vi "GenerateCode.vi"(1 "Terms":T1[](array[typedef]), 3 "Diagram":refnum<vi>, 5 "XRef":refnum<vi>, 6 "State In":T4) -> (0 "Generated Code?":bool, 2 "State Out":T4, 4 "Reply":string[](array[string]))   [LabVIEW 2015, in "Async.xnode"]
doc: "This ability VI is called when it is time to define the execution behavior of your XNode via LabVIEW's scripting API. This VI is only called when you have previously informed LabVIEW that you need to script through a GenerateCode reply. Diagram is a reference to a diagram of a temporary VI. This diagram contains exactly one front panel terminal for each terminal of your XNode. Terms is an array of pairs of Term IDs and terminal references. LabVIEW will copy code scripted into this diagram into your XNode and connect everything to the correct terminals. The front panel terminals that are on this diagram are special in that they can only be on the top level diagram.\n \n Generate Code? is used to tell LabVIEW whether or not you want to copy the scripted diagram over. If there is an error and you wish not to commit the changes, then the old XNode behavior will be left unchanged. If you set Generate Code? to false, then this VI will be called again next time type propagation is run. Otherwise, it will not be called until you indicate that it should be through the reply on another ability VI.\n \n Because the diagram you are scripting into is separate from the VI containing the XNode instance, type propagation and the data manager will run on the temporary VI after each scripting call.\n \n You should not use the Copy scripting method to move code into the temporary VI. This will adversely affect the user's clipboard. You should use the Move scripting method instead.\n\nDefault behavior: None.\n\nThis ability does not provide UI and OS messages are not handled.\n\nSee also: ModifyCode"
uses:
  Async.xnode
  State.ctl
  <vilib>/Utility/miscctls.llb/LVRectTypeDef.ctl
  <vilib>/picture/picture.llb/imagedata.ctl
  <vilib>/XNodeSupport/XNodeTermIDPair.ctl
  <vilib>/XNodeSupport/XNodeTermRef.ctl
  <vilib>/XNodeSupport/XNodeString.ctl
  <vilib>/Erdos Miller/LV-Scripting/LV-Scripting.lvlib
  <vilib>/Erdos Miller/LV-VI/LV-VI.lvlib
  <vilib>/XNodeSupport/NI_XNodeSupport.lvlib
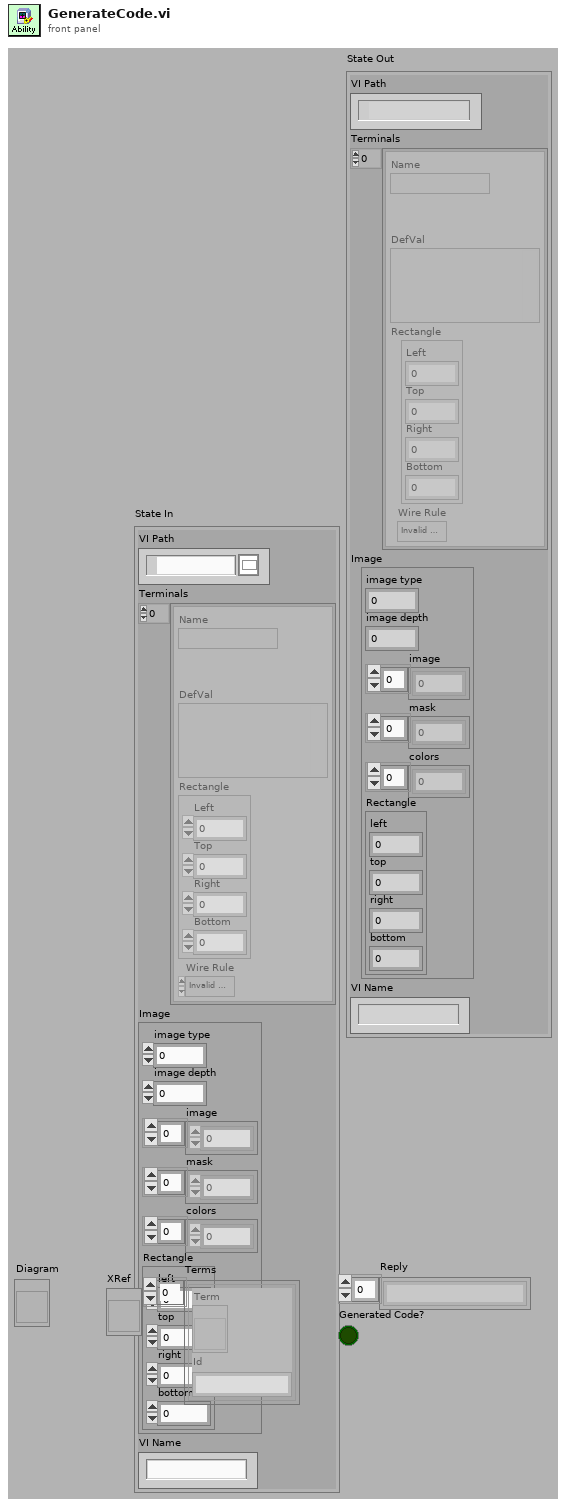
[diagram p1: front panel]
types:
  T1 = typedef "NI_XNodeSupport.lvlib/XNodeTermIDPair.ctl" = cluster{"Term":T2, "Id":T3}
  T2 = typedef "NI_XNodeSupport.lvlib/XNodeTermRef.ctl" = refnum<vi>
  T3 = typedef "NI_XNodeSupport.lvlib/XNodeString.ctl" = string
  T4 = typedef "Async.xnode/State.ctl" = cluster{"VI Path":path, "Terminals":cluster{"Name":string, "DefVal":variant, "Rectangle":T5, "Wire Rule":enum16{"Invalid Wire Rule", "Required", "Recommended", "Optional", "Dynamic Dispatch"}}[], "Image":T6, "VI Name":string}
  T5 = typedef "LVRectTypeDef.ctl" = cluster{"Left":i16, "Top":i16, "Right":i16, "Bottom":i16}
  T6 = typedef "imagedata.ctl" = cluster{"image type":i32, "image depth":i32, "image":u8[], "mask":u8[], "colors":u32[], "Rectangle":cluster{"left":i16, "top":i16, "right":i16, "bottom":i16}}
  T7 = cluster{"Name":string, "DefVal":variant, "Rectangle":T5, "Wire Rule":enum16{"Invalid Wire Rule", "Required", "Recommended", "Optional", "Dynamic Dispatch"}}[]
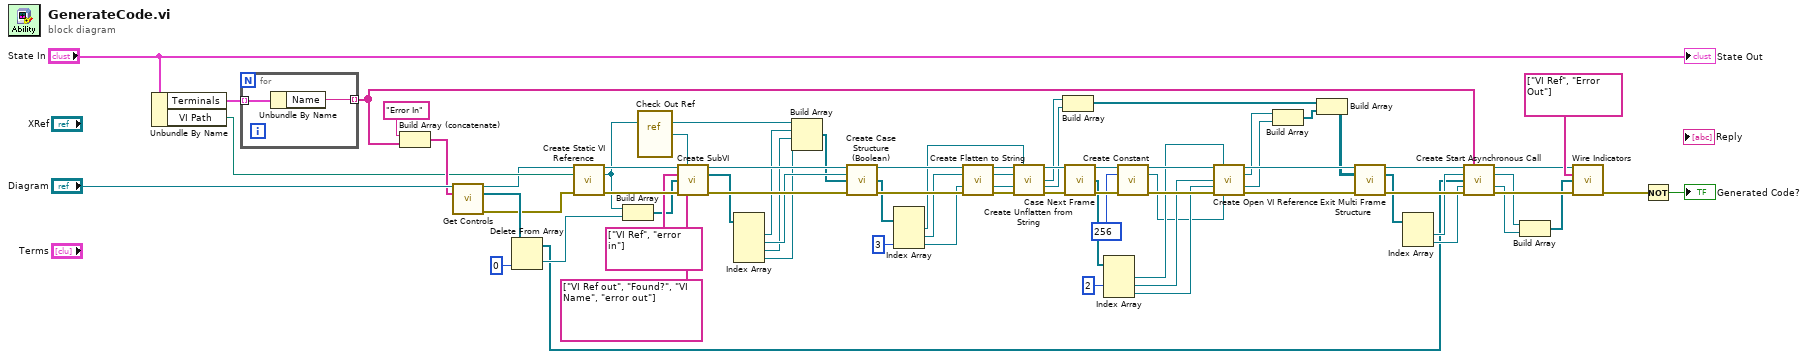
[diagram p0: block diagram]
diagram:
  n1 = Unbundle By Name("State In") -> ("Terminals"=w72:T7, "VI Path"=w67:path)
  n2 = for {
    tunnel: w72 -> [w76] mode=indexing
    tunnel: [w75] -> w4 mode=indexing
    n3 = Unbundle By Name(w76) -> ("Name"=w75:string)
  }
  n4 = Build Array (concatenate)("Error In" ("string"), w4) -> (w70:string[])
  n5 = call <vilib>:"Get Controls.vi"("Diagram in"="Diagram", "Control Names"=w70) -> ("Diagram out"=w66:refnum<vi>, "Control Terminals"=w69:refnum<vi>[], "error out"=w65:errorcluster)  [unwired: 11 in]
  n6 = Delete From Array(array=w69, index=0) -> (deleted portion=w59:refnum<vi>, array with subset deleted=w5:refnum<vi>[])  [unwired: 1 in]
  n7 = call <vilib>:"Create Static VI Reference.vi"("Diagram in"=w66, "VI Path"=w67, "error in (no error)"=w65) -> ("Diagram out"=w62:refnum<vi>, "Terminal"=w52:refnum<vi>, "error out"=w61:errorcluster)  [unwired: 10 in]
  n8 = Build Array(w52, w59) -> (w58:refnum<vi>[])
  n9 = vi-ref <vilib>:"Check Out Ref.vi"() -> (w63:refnum<vi>)
  n10 = call <vilib>:"Create SubVI.vi"("Diagram in"=w62, "VI Reference"=w63, "Input Names"=string[] ["VI Ref", "error in"], "Inputs"=w58, "Output Names"=string[] ["VI Ref out", "Found?", "VI Name", "error out"], "error in (no error)"=w61) -> ("Diagram out"=w55:refnum<vi>, "Outputs"=w54:refnum<vi>[], "error out"=w56:errorcluster)  [unwired: 7 in]
  n11 = Index Array(array=w54) -> (element #1=w51:refnum<vi>, element #2=w53:refnum<vi>, element #3=w50:refnum<vi>, element #4=w34:refnum<vi>)  [unwired: 4 in]
  n12 = Build Array(w52, w51, w50, w34) -> (w49:refnum<vi>[])
  n13 = call <vilib>:"Create Case Structure (Boolean).vi"("Diagram in"=w55, "Selector"=w53, "Inputs"=w49, "error in (no error)"=w56) -> ("Selected Diagram"=w48:refnum<vi>, "Inputs"=w46:refnum<vi>[], "error out"=w47:errorcluster)  [unwired: 8 in, 1 out]
  n14 = Index Array(array=w46, index #3=3 ("index")) -> (element #1=w40:refnum<vi>, element #2=w45:refnum<vi>, element #3=w33:refnum<vi>)  [unwired: 2 in]
  n15 = call <vilib>:"Create Flatten to String.vi"("Diagram in"=w48, "anything"=w45, "error in"=w33, "error in (no error)"=w47) -> ("Diagram out"=w44:refnum<vi>, "data string"=w42:refnum<vi>, 10:"error out"=w41:refnum<vi>, 15:"error out"=w43:errorcluster)  [unwired: 8 in]
  n16 = call <vilib>:"Create Unflatten from String.vi"("Diagram in"=w44, "type"=w40, "binary string"=w42, "error in"=w41, "error in (no error)"=w43) -> ("Diagram out"=w39:refnum<vi>, "value"=w21:refnum<vi>, 10:"error out"=w20:refnum<vi>, 15:"error out"=w38:errorcluster)  [unwired: 6 in, 1 out]
  n17 = Build Array(w21, w20) -> (w17:refnum<vi>[])
  n18 = call <vilib>:"Case Next Frame.vi"("Diagram in"=w39, "error in (no error)"=w38) -> ("Selected Diagram"=w37:refnum<vi>, "Inputs"=w31:refnum<vi>[], "error out"=w36:errorcluster)  [unwired: 10 in, 1 out]
  n19 = Index Array(array=w31, index #2=2 ("index")) -> (element #1=w27:refnum<vi>, element #2=w26:refnum<vi>, element #3=w25:refnum<vi>)  [unwired: 2 in]
  n20 = call <vilib>:"Create Constant.vi"("Diagram in"=w37, "Type"=256, "error in (no error)"=w36) -> ("Diagram out"=w29:refnum<vi>, "Terminal"=w24:refnum<vi>, "error out"=w28:errorcluster)  [unwired: 10 in]
  n21 = call <vilib>:"Create Open VI Reference.vi"("Diagram in"=w29, "type specifier"=w27, "vi path"=w26, "error in"=w25, "error in (no error)"=w28, "options"=w24) -> ("Diagram out"=w23:refnum<vi>, "vi reference"=w19:refnum<vi>, 10:"error out"=w18:refnum<vi>, 15:"error out"=w22:errorcluster)  [unwired: 6 in]
  n22 = Build Array(w19, w18) -> (w16:refnum<vi>[])
  n23 = Build Array(w17, w16) -> (w15:refnum<vi>[][])
  n24 = call <vilib>:"Exit Multi Frame Structure.vi"("Diagram in"=w23, "Outputs"=w15, "error in (no error)"=w22) -> ("Diagram out"=w9:refnum<vi>, "Outputs"=w13:refnum<vi>[], "error out"=w14:errorcluster)  [unwired: 10 in]
  n25 = Index Array(array=w13) -> (element #1=w7:refnum<vi>, element #2=w6:refnum<vi>)  [unwired: 2 in]
  n26 = call <vilib>:"Create Start Asynchronous Call.vi"("Diagram in"=w9, "Input Names"=w4, "reference"=w7, "Inputs"=w5, "error in"=w6, "error in (no error)"=w14) -> ("Diagram out"=w8:refnum<vi>, "reference out"=w3:refnum<vi>, 10:"error out"=w2:refnum<vi>, 15:"error out"=w10:errorcluster)  [unwired: 6 in]
  n27 = Build Array(w3, w2) -> (w1:refnum<vi>[])
  n28 = call <vilib>:"Wire Indicators.vi"("Diagram in"=w8, "Indicator Names"=string[] ["VI Ref", "Error Out"], "Outputs"=w1, "error in (no error)"=w10) -> ("error out"=w11:errorcluster)  [unwired: 10 in, 1 out]
  n29 = Not(x=w11) -> (.not. x?=→"Generated Code?":bool)
  "State Out" <- "State In"
